vi "ini_sesion.vi"(8 "error in (no error)":errorcluster, 11 "p2p vst in":refnum<class "p2p vst.lvclass">) -> (0 "error out":errorcluster, 3 "p2p vst out":refnum<class "p2p vst.lvclass">)   [LabVIEW 2021, in "p2p vst.lvclass"]
uses:
  p2p vst.lvclass
  p2p vst.lvclass/p2p vst.ctl
  <instrlib>/niRFSG/niRFSG.llb/niRFSG Ref Clock Sources.ctl
  <instrlib>/niRFSG/niRFSG.llb/niRFSG Stream Endpoint Names.ctl
  <instrlib>/niRFSG/niRFSG.llb/niRFSG Configure Start Trigger P2P Endpoint Fullness.vi
  <vilib>/FPGAPlugInAG/PXIe-6592R/niLvFpga_Open_PXIe-6592R.vi
  <vilib>/rvi/interface/common/dynamic/niFpgaDynamicAddResources.vi
  <vilib>/FPGAPlugInAG/Dynamic/niLvFpga_P2PGetEndpoint_Dynamic.vi
  <vilib>/FPGAPlugInAG/PXIe-5785 (KU060)/niLvFpga_Open_PXIe-5785 (KU060).vi
  <vilib>/FPGAPlugInAG/PXIe-7915/niLvFpga_Open_PXIe-7915.vi
  <vilib>/Utility/error.llb/Error Cluster From Error Code.vi
  <vilib>/rvi/interface/common/niFpgaWaitOnOcc.vi
  <vilib>/rvi/errors/niLvFpgaAdjustHostInterfaceError.vi
  <vilib>/rvi/interface/nirviOpenFPGA/nirviOpenFPGA.xnode
  FPGA Bitfiles/6592R_p2p_IQ_gen_1_6GHz_max.lvbitx
  <vilib>/rvi/interface/nirviMethod/nirviMethod.xnode
  FPGA Bitfiles/5785_p2p_IQ_gen_1_92GHz_8+4.lvbitx
  FPGA Bitfiles/5785_Multi_Emitter_p2p_IQ_gen_1_6GHz.lvbitx
  <vilib>/rvi/interface/nirviReadWriteControl/nirviReadWriteControl.xnode
  <vilib>/rvi/errors/niLvFpgaMergeErrorWithErrorCode.vi
  <vilib>/FPGAPlugInAG/Dynamic/niLvFpga_StopFifo_Dynamic.vi
  <vilib>/FPGAPlugInAG/Dynamic/niLvFpga_ConfigureFifo_Dynamic.vi
  NiFpgaLv.dll
  <vilib>/rvi/interface/Simulation/niFpgaSimulationCallBeginRW.vi
  FPGA Bitfiles/5785_Multi_Emitter_p2p_IQ_gen_3.2GHz_max.lvbitx
  FPGA Bitfiles/7915_p2p_IQ_gen_1_92GHz_8+4.lvbitx
  FPGA Bitfiles/7915_p2p_IQ_gen_3_2GHz_max.lvbitx
  FPGA Bitfiles/7915_p2p_IQ_gen_1_6GHz_max.lvbitx
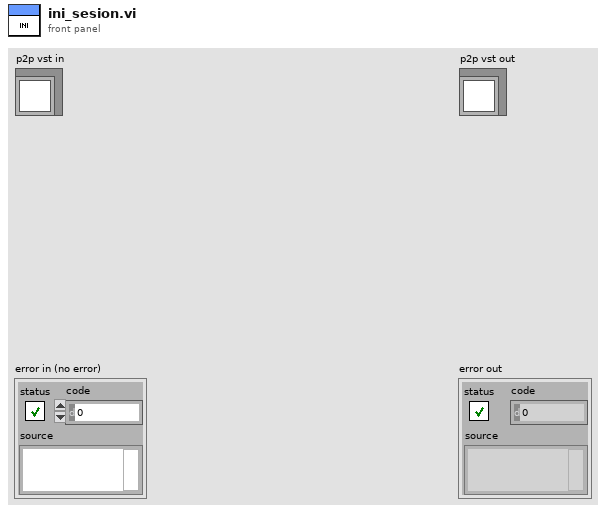
[diagram p1: front panel]
types:
  T1 = typedef "nirio_resource_hc.ctl" = tag
  T2 = typedef "niRFSG Ref Clock Sources.ctl" = string
  T3 = typedef "niRFSG Stream Endpoint Names.ctl" = string
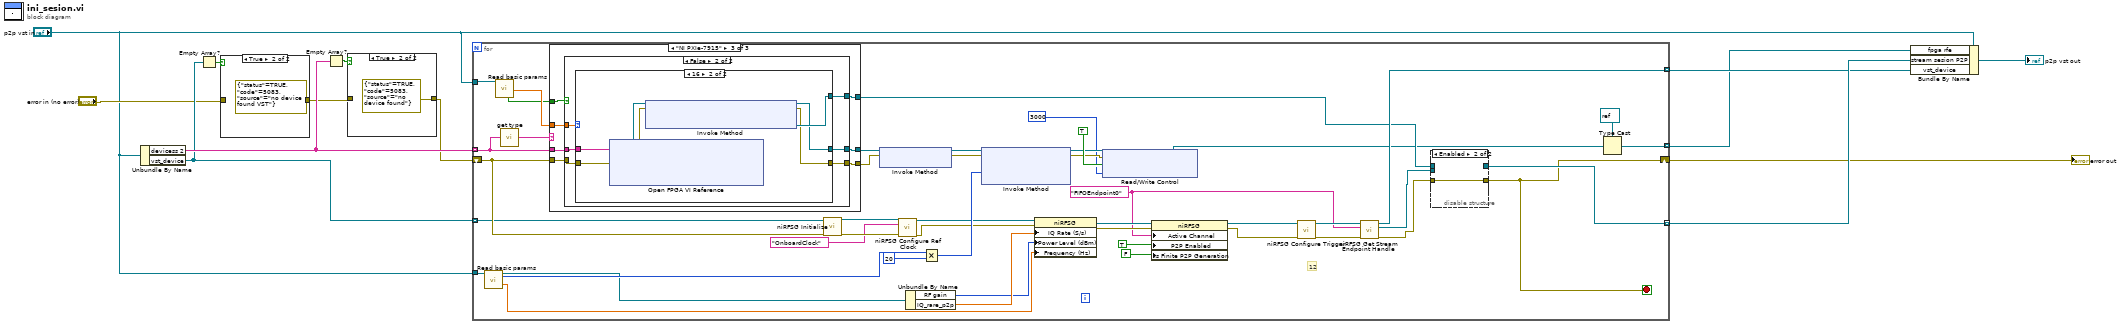
[diagram p0: block diagram]
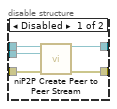
[diagram p4: hidden frame]
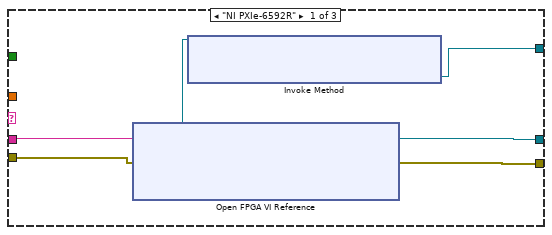
[diagram p5: hidden frame]
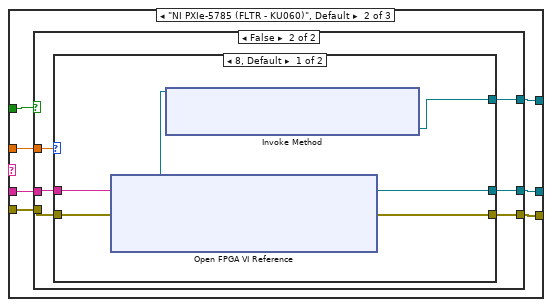
[diagram p6: hidden frame]
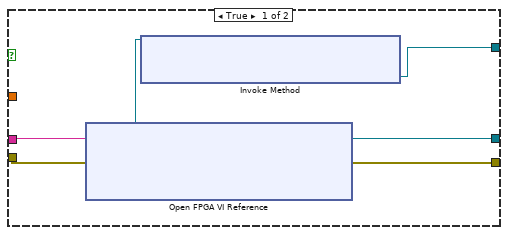
[diagram p7: hidden frame]
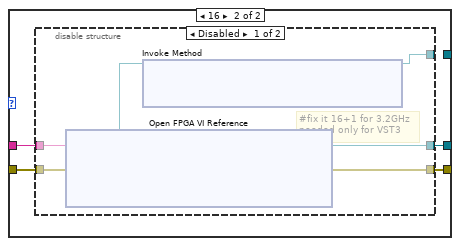
[diagram p8: hidden frame]
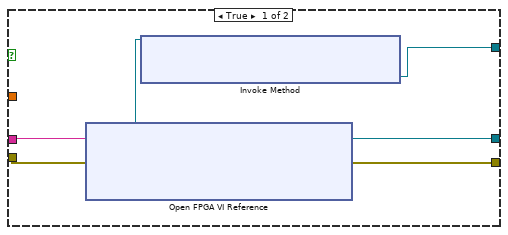
[diagram p10: hidden frame]
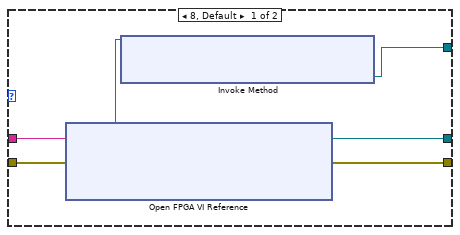
[diagram p11: hidden frame]
diagram:
  n1 = Unbundle By Name("p2p vst in") -> ("devicess 2"=w11:T1[], "vst_device"=w9:refnum<k15>[])
  n2 = Empty Array?(array=w9) -> (empty?=w10:bool)
  n3 = case shown="True" w10 {
    tunnel: [w14 errorcluster {"status"=TRUE, "code"=5083, "source"="no device found VST"} ("error in (no error)")] -> w8
    tunnel: "error in (no error)" -> [w14 _]
    frame False {
    }
    frame True {
    }
  }
  n4 = Empty Array?(array=w11) -> (empty?=w12:bool)
  n5 = case shown="True" w12 {
    tunnel: [w16 errorcluster {"status"=TRUE, "code"=5083, "source"="no device found"} ("error in (no error)")] -> w7
    tunnel: w8 -> [w16 _]
    frame False {
    }
    frame True {
    }
  }
  n6 = for {
    tunnel: [w32] -> w2 mode=indexing
    shift-right: [w25] -> w4
    shift-left: w7 -> [w52]
    tunnel: w11 -> [w29] mode=indexing
    tunnel: w9 -> [w49] mode=indexing
    tunnel: [w48] -> w13 mode=indexing
    tunnel: "p2p vst in" -> [w38]
    tunnel: [w40] -> w3 mode=indexing
    tunnel: "p2p vst in" -> [w31]
    stop <- w25 stop-if-true
    w18 = T3 "FIFOEndpoint0" ("stream endpoint")
    # "12"
    n7 = call-dynamic "Read basic params.vi"("device_type in"=w38) -> ("device_type out"=w36:refnum<class "p2p vst.lvclass">, "buffer size"=w37:u32, "center frequency (Hz)"=w19:dbl)  [unwired: 11 in, 5 out]
    n8 = call-dynamic "Read basic params.vi"("device_type in"=w31) -> ("use arb files"=w27:bool, "SPC"=w30:dbl)  [unwired: 11 in, 6 out]
    n9 = call "get type.vi"("RIO Device"=w29) -> ("Product Name"=w28:string)
    n10 = case shown="\"NI PXIe-7915\"" w28 {
      tunnel: [w72 w81 w113] -> w61
      tunnel: w52 -> [w73 w80 w112]
      tunnel: [w71 w79 w111] -> w50
      tunnel: [w70 w78 w110] -> w35
      tunnel: w30 -> [_ w77 w109]
      tunnel: w29 -> [w74 w76 w108]
      tunnel: w27 -> [_ w75 w107]
      frame "NI PXIe-6592R" {
        n11 = xnode "Open FPGA VI Reference"("error in"=w73, "resource name"=w74) -> ("FPGA VI Reference Out"=w71:refnum<k20>, "error out"=w72:errorcluster)
        n12 = xnode "Invoke Method"("FPGA VI Reference In"=w71) -> ("Writer"=w70:refnum<k20>)  [unwired: 1 in, 2 out]
      }
      frame "NI PXIe-5785 (FLTR - KU060)", Default {
        n13 = case shown="False" w75 {
          tunnel: [w86 w92] -> w81
          tunnel: w80 -> [w85 w91]
          tunnel: [w84 w90] -> w79
          tunnel: [w83 w89] -> w78
          tunnel: w77 -> [_ w88]
          tunnel: w76 -> [w82 w87]
          frame True {
            n14 = xnode "Open FPGA VI Reference"("error in"=w85, "resource name"=w82) -> ("FPGA VI Reference Out"=w84:refnum<k20>, "error out"=w86:errorcluster)
            n15 = xnode "Invoke Method"("FPGA VI Reference In"=w84) -> ("Writer"=w83:refnum<k20>)  [unwired: 1 in, 2 out]
          }
          frame False {
            n16 = case shown="8, Default" w88 {
              tunnel: [w97 w101] -> w92
              tunnel: w87 -> [w96 w100]
              tunnel: w91 -> [w95 w99]
              tunnel: [w94 w98] -> w90
              tunnel: [w93 _] -> w89
              frame 8, Default {
                n17 = xnode "Open FPGA VI Reference"("error in"=w95, "resource name"=w96) -> ("FPGA VI Reference Out"=w94:refnum<k20>, "error out"=w97:errorcluster)
                n18 = xnode "Invoke Method"("FPGA VI Reference In"=w94) -> ("Writer"=w93:refnum<k20>)  [unwired: 1 in, 2 out]
              }
              frame 16 {
                n19 = disable-structure shown="Disabled" {
                  disable-tunnel: [w106 _] -> w101
                  disable-tunnel: w100 -> [w105 _]
                  disable-tunnel: w99 -> [w104 _]
                  disable-tunnel: [w103 _] -> w98
                  disable-tunnel: [w102 _] -> _
                  frame Disabled {
                    # "#fix it 16+1 for 3.2GHz\nneeded only for VST3"
                    n20 = xnode "Open FPGA VI Reference"("error in"=w104, "resource name"=w105) -> ("FPGA VI Reference Out"=w103:refnum<k20>, "error out"=w106:errorcluster)
                    n21 = xnode "Invoke Method"("FPGA VI Reference In"=w103) -> ("FPGA VI Reference Out"=w102:refnum<k20>)  [unwired: 1 in, 2 out]
                  }
                  frame Enabled {
                  }
                }
              }
            }
          }
        }
      }
      frame "NI PXIe-7915" {
        n22 = case shown="False" w107 {
          tunnel: [w118 w124] -> w113
          tunnel: w112 -> [w117 w123]
          tunnel: [w116 w122] -> w111
          tunnel: [w115 w121] -> w110
          tunnel: w109 -> [_ w120]
          tunnel: w108 -> [w114 w119]
          frame True {
            n23 = xnode "Open FPGA VI Reference"("error in"=w117, "resource name"=w114) -> ("FPGA VI Reference Out"=w116:refnum<k20>, "error out"=w118:errorcluster)
            n24 = xnode "Invoke Method"("FPGA VI Reference In"=w116) -> ("Writer"=w115:refnum<k20>)  [unwired: 1 in, 2 out]
          }
          frame False {
            n25 = case shown="16" w120 {
              tunnel: [w129 w130] -> w124
              tunnel: w119 -> [w128 w136]
              tunnel: w123 -> [w127 w135]
              tunnel: [w126 w132] -> w122
              tunnel: [w125 w133] -> w121
              frame 8, Default {
                n26 = xnode "Open FPGA VI Reference"("error in"=w127, "resource name"=w128) -> ("FPGA VI Reference Out"=w126:refnum<k20>, "error out"=w129:errorcluster)
                n27 = xnode "Invoke Method"("FPGA VI Reference In"=w126) -> ("Writer"=w125:refnum<k20>)  [unwired: 1 in, 2 out]
              }
              frame 16 {
                n28 = xnode "Open FPGA VI Reference"("error in"=w135, "resource name"=w136) -> ("FPGA VI Reference Out"=w134:refnum<k20>, "error out"=w131:errorcluster)
                n29 = xnode "Invoke Method"("FPGA VI Reference In"=w134, "error in"=w131) -> ("FPGA VI Reference Out"=w132:refnum<k20>, "error out"=w130:errorcluster, "Writer"=w133:refnum<k20>)
              }
            }
          }
        }
      }
    }
    n30 = call <instrlib>:"niRFSG Initialize.vi"("resource name"=w49, "error in"=w52) -> ("instrument handle"=w55:refnum<k15>, "error out"=w54:errorcluster)  [unwired: 12 in]
    n31 = xnode "Invoke Method"("FPGA VI Reference In"=w50, "error in"=w61) -> ("FPGA VI Reference Out"=w59:refnum<k20>, "error out"=w60:errorcluster)
    n32 = call <instrlib>:"niRFSG Configure Ref Clock.vi"("instrument handle"=w55, "ref clock source"=T2 "OnboardClock", "error in"=w54) -> ("instrument handle out"=w45:refnum<k15>, "error out"=w44:errorcluster)  [unwired: 11 in]
    n33 = Unbundle By Name(w36) -> ("RF gain"=w20:i32, "IQ_rare_p2p"=w41:dbl)
    n34 = Multiply(x=w37, y=u32 20) -> (x*y=w63:u32)
    n35 = xnode "Invoke Method"("FPGA VI Reference In"=w59, "error in"=w60, "Requested Depth"=w63) -> ("FPGA VI Reference Out"=w57:refnum<k20>, "error out"=w56:errorcluster)  [unwired: 1 out]
    n36 = property class="niRFSG"(reference=w45, error in=w44, "IQ Rate (S/s)"=w41, "Power Level (dBm)"=w20, "Frequency (Hz)"=w19) -> (reference out=w43:refnum<k15>, error out=w42:errorcluster)
    n37 = xnode "Read/Write Control"("FPGA VI Reference In"=w57, "error in"=w56, "reset system clock"=TRUE, "P2P empty room for runing"=u32 3000) -> ("FPGA VI Reference Out"=w34:refnum<k20>)  [unwired: 1 out]
    n38 = property class="niRFSG"(reference=w43, error in=w42, "Active Channel"=w18, "P2P Enabled"=TRUE ("Peer-to-Peer:Enabled"), "Is Finite P2P Generation"=FALSE ("Peer-to-Peer:Is Finite Generation")) -> (reference out=w24:refnum<k15>, error out=w23:errorcluster)
    n39 = call-poly <instrlib>:"niRFSG Configure Trigger.vi"("instrument handle"=w24, "error in"=w23) -> ("instrument handle out"=w22:refnum<k15>, "error out"=w21:errorcluster)  [unwired: 12 in]
    n40 = call <instrlib>:"niRFSG Get Stream Endpoint Handle.vi"("instrument handle"=w22, "stream endpoint"=w18, "error in"=w21) -> ("instrument handle out"=w40:refnum<k15>, "reader handle"=w51:refnum<k20>, "error out"=w26:errorcluster)  [unwired: 10 in]
    n41 = disable-structure shown="Enabled" {
      disable-tunnel: w51 -> [w68 _]
      disable-tunnel: [w67 _] -> w48
      disable-tunnel: w35 -> [w66 _]
      disable-tunnel: w26 -> [w65 w69]
      disable-tunnel: [w64 w69] -> w25
      frame Disabled {
        n42 = call <vilib>:"niP2P Create Peer to Peer Stream.vi"("writer"=w66, "reader"=w68, "error in (no error)"=w65) -> ("stream session"=w67:refnum<k20>, "error out"=w64:errorcluster)  [unwired: 11 in]
      }
      frame Enabled {
      }
    }
    n43 = Type Cast(type=refnum<k20> refnum ("FPGA VI Reference Out"), x=w34) -> (*(type *) &x=w32:refnum<k20>)
  }
  "error out" <- w4
  n44 = Bundle By Name(cluster="p2p vst in", "fpga rfe"=w2, "stream sesion P2P"=w13, "vst_device"=w3) -> (→"p2p vst out":refnum<class "p2p vst.lvclass">)
